vi "svl_Set Input Coupling and IEPE Excitation (Active Ch).vi"(0 "AI task name":refnum<k21>, 5 "active channels":refnum<k21>, 7 "DSA channel settings":T1={"coupling"=10045, "enable excitation"=FALSE, "excitation value"=4.0} {"excitation value" format="%.1f"; "coupling" items=["AC"=10045, "DC"=10050, "GND"=10066]}, 9 "time to settle [s]":dbl, 11 "error in (no error)":errorcluster) -> (4 "dup AI task name":refnum<k21>, 15 "error out":errorcluster)   [LabVIEW 2017]
uses:
  <resource>/objmgr/daqmx.rc
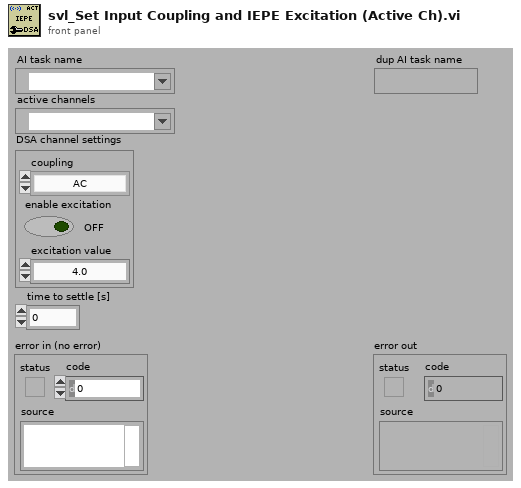
[diagram p1: front panel]
types:
  T1 = cluster{"coupling":i32, "enable excitation":bool, "excitation value":dbl}
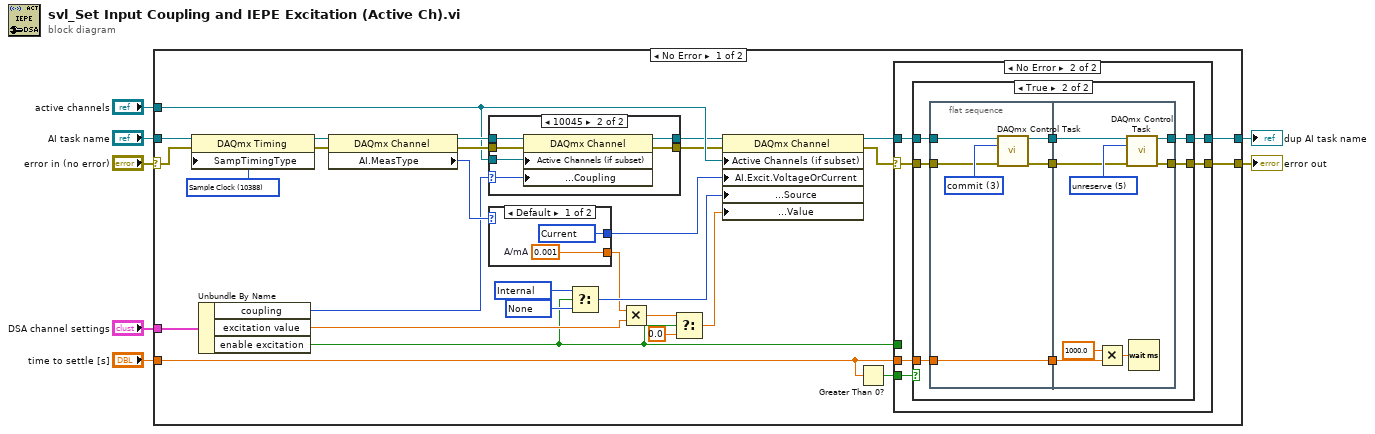
[diagram p0: block diagram]
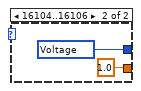
[diagram p2: hidden frame]
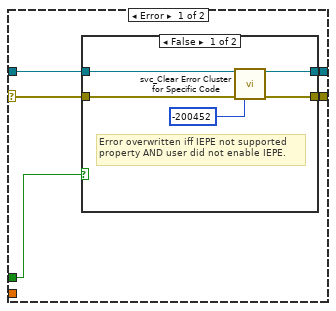
[diagram p4: hidden frame]
diagram:
  n1 = case shown="No Error" "error in (no error)" {
    selector: "error in (no error)" -> [w24 w90]
    tunnel: "AI task name" -> [w25 w91]
    tunnel: [w36 w90] -> w2
    tunnel: [w35 w91] -> w3
    tunnel: "time to settle [s]" -> [w34 _]
    tunnel: "DSA channel settings" -> [w33 _]
    tunnel: "active channels" -> [w11 _]
    frame No Error {
      w21 = 10230 items=["Internal"=10200, "External"=10167, "None"=10230] ("AI.Excit.Src")
      w23 = 10388 items=["Sample Clock"=10388, "Burst Handshake"=12548, "Handshake"=10389, "Implicit"=10451, "On Demand"=10390, "Change Detection"=12504, "Pipelined Sample Clock"=14668] ("SampTimingType")
      w22 = 10200 items=["Internal"=10200, "External"=10167, "None"=10230] ("AI.Excit.Src")
      n2 = property class="DAQmx Timing"(reference=w25, error in=w24, "SampTimingType"=w23) -> (reference out=w15:refnum<k21>, error out=w14:errorcluster)
      n3 = Unbundle By Name(w33) -> ("coupling"=w10:i32, "excitation value"=w30:dbl, "enable excitation"=w17:bool)
      n4 = property class="DAQmx Channel"(reference=w15, error in=w14) -> (reference out=w13:refnum<k21>, error out=w12:errorcluster, "AI.MeasType"=w19:i32)
      n5 = case shown="10045" w10 {
        selector: w10 -> [_ w43]
        tunnel: [w42 w48] -> w9
        tunnel: w12 -> [w41 w47]
        tunnel: [w41 w46] -> w8
        tunnel: w13 -> [w42 w45]
        tunnel: w11 -> [_ w44]
        frame Default {
        }
        frame 10045 {
          n6 = property class="DAQmx Channel"(reference=w45, error in=w47, "Active Channels (if subset)"=w44, "Analog Input:General Properties:Input Configuration:Coupling"=w43) -> (reference out=w48:refnum<k21>, error out=w46:errorcluster)
        }
      }
      n7 = case shown="Default" w19 {
        tunnel: [w38 w40] -> w18
        tunnel: [w37 1.0 ("A/mA")] -> w16
        frame Default {
          w37 = 0.001  # A/mA
          w38 = 10134 items=["Voltage"=10322, "Current"=10134] ("AI.Excit.VoltageOrCurrent")
        }
        frame 16104..16106 {
          w40 = 10322 items=["Voltage"=10322, "Current"=10134] ("AI.Excit.VoltageOrCurrent")
        }
      }
      n8 = Select(t=w22, s=w17, f=w21) -> (s? t:f=w20:i32)
      n9 = Multiply(x=w16, y=w30) -> (x*y=w28:dbl)
      n10 = Select(t=w28, s=w17, f=0.0) -> (s? t:f=w27:dbl)
      n11 = property class="DAQmx Channel"(reference=w9, error in=w8, "Active Channels (if subset)"=w11, "AI.Excit.VoltageOrCurrent"=w18, "Analog Input:General Properties:Signal Conditioning:Excitation:Source"=w20, "Analog Input:General Properties:Signal Conditioning:Excitation:Value"=w27) -> (reference out=w32:refnum<k21>, error out=w26:errorcluster)
      n12 = Greater Than 0?(x=w34) -> (x > 0?=w31:bool)
      n13 = case shown="No Error" w26 {
        selector: w26 -> [w49 w60]
        tunnel: [w50 w65] -> w36
        tunnel: [w51 w64] -> w35
        tunnel: w34 -> [_ w63]
        tunnel: w32 -> [w52 w62]
        tunnel: w31 -> [_ w61]
        tunnel: w17 -> [w53 _]
        frame Error {
          n14 = case shown="False" w53 {
            tunnel: [w57 w59] -> w51
            tunnel: w52 -> [w57 w59]
            tunnel: [w55 w58] -> w50
            tunnel: w49 -> [w56 w58]
            frame False {
              # "Error overwritten iff IEPE not supported\nproperty AND user did not enable IEPE."
              n15 = call <vilib>:"svc_Clear Error Cluster for Specific Code.vi"("error in (no error)"=w56, "code"=-200452) -> ("error out"=w55:errorcluster)  [unwired: 12 in, 1 out]
            }
            frame True {
              # "If the user enables IEPE on a device\nthat does not supprt it, DAQmx error\nis propagated."
            }
          }
        }
        frame No Error {
          n16 = case shown="True" w61 {
            tunnel: [w67 w75] -> w64
            tunnel: [w66 w74] -> w65
            tunnel: w63 -> [_ w70]
            tunnel: w62 -> [w67 w69]
            tunnel: w60 -> [w66 w68]
            frame False {
            }
            frame True {
              n17 = flat-sequence {
                tunnel: [w81] -> w73
                tunnel: [w80] -> w72
                tunnel: [w78] -> w71
                tunnel: w70 -> [w78]
                tunnel: w69 -> [w77]
                tunnel: w68 -> [w76]
                tunnel: [w84] -> w74
                tunnel: [w85] -> w75
                tunnel: w73 -> [w82]
                tunnel: w72 -> [w83]
                tunnel: w71 -> [w88]
                frame #0 {
                  w79 = 3 items=["verify"=2, "reserve"=4, "commit"=3, "unreserve"=5, "abort"=6] ("action")
                  n18 = call <vilib>:"DAQmx Control Task.vi"("task/channels in"=w77, "action"=w79, "error in"=w76) -> ("task out"=w81:refnum<k21>, "error out"=w80:errorcluster)  [unwired: 11 in]
                }
                frame #1 {
                  w86 = 5 items=["verify"=2, "reserve"=4, "commit"=3, "unreserve"=5, "abort"=6] ("action")
                  n19 = Multiply(x=1000.0 ("y"), y=w88) -> (x*y=w89:dbl)
                  n20 = call <vilib>:"DAQmx Control Task.vi"("task/channels in"=w82, "action"=w86, "error in"=w83) -> ("task out"=w85:refnum<k21>, "error out"=w84:errorcluster)  [unwired: 11 in]
                  n21 = Wait (ms)(milliseconds to wait=w89) -> ()  [unwired: 1 out]
                }
              }
            }
          }
        }
      }
    }
    frame Error {
    }
  }
  "error out" <- w2
  "dup AI task name" <- w3
